vi "AppMenuSelection.vi"(8 "error in (no error)":errorcluster, 10 "Menu Selection in":string, 11 "xceRootNode in":refnum<class "xceRootNode.lvclass">) -> (0 "error out":errorcluster, 1 "New Message":string, 2 "Menu Selection out":string, 3 "xceRootNode out":refnum<class "xceRootNode.lvclass">)   [LabVIEW 2013, in "xceRootNode.lvclass"]
doc: "Processes the action related to the application level menu selection. For instance used when the user chooses \"File->Save\""
uses:
  xceRootNode.lvclass
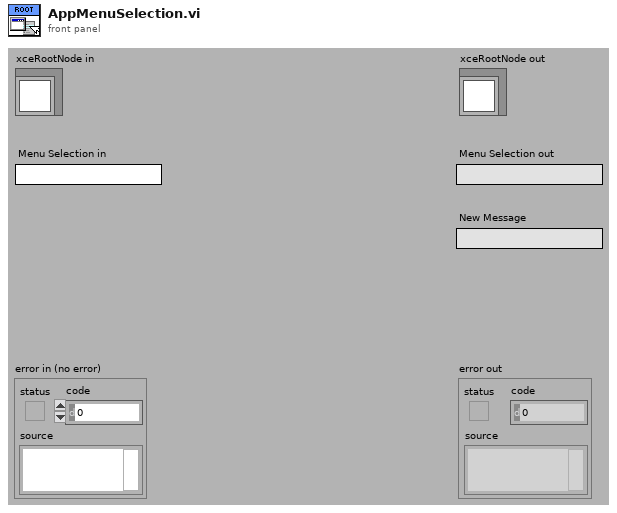
[diagram p1: front panel]
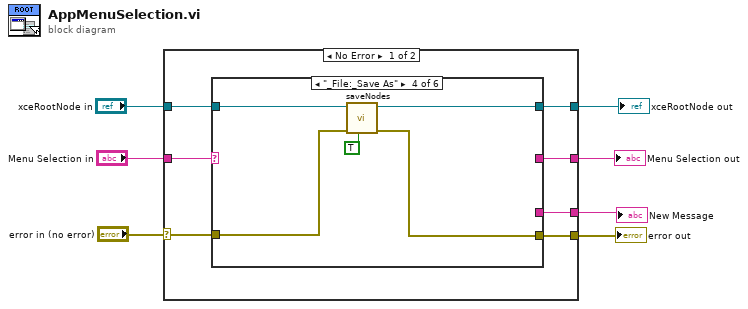
[diagram p0: block diagram]
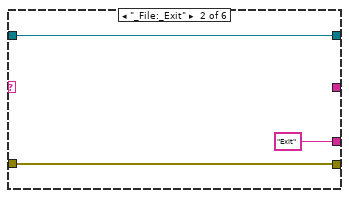
[diagram p3: hidden frame]
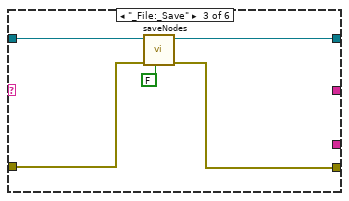
[diagram p4: hidden frame]
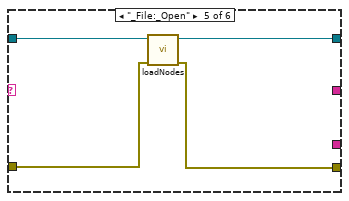
[diagram p5: hidden frame]
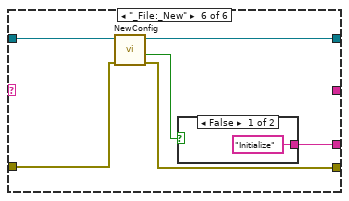
[diagram p6: hidden frame]
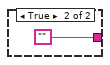
[diagram p7: hidden frame]
diagram:
  n1 = case shown="No Error" "error in (no error)" {
    selector: "error in (no error)" -> [w9 w44]
    tunnel: [w8 w44] -> w6
    tunnel: [w10 w43] -> w4
    tunnel: "xceRootNode in" -> [w11 w43]
    tunnel: "Menu Selection in" -> [w14 _]
    tunnel: [w13 _] -> w2
    tunnel: [w12 _] -> w1
    frame No Error {
      n2 = case shown="\"_File:_Save As\"" w14 {
        selector: w14 -> [w17 _ _ _ _ _]
        tunnel: [_ "Exit" _ _ _ w36] -> w13
        tunnel: [w17 _ _ _ _ _] -> w12
        tunnel: w11 -> [w15 w19 w25 w30 w34 w40]
        tunnel: [w15 w19 w24 w29 w33 w39] -> w10
        tunnel: w9 -> [w16 w18 w23 w28 w32 w38]
        tunnel: [w16 w18 w22 w27 w31 w35] -> w8
        frame Default {
        }
        frame "_File:_Exit" {
        }
        frame "_File:_Save" {
          n3 = call "saveNodes.vi"("Save As"=FALSE, "error in (no error)"=w23, "xceRootNode in"=w25) -> ("error out"=w22:errorcluster, "xceRootNode out"=w24:refnum<class "xceRootNode.lvclass">)  [unwired: 6 in, 1 out]
        }
        frame "_File:_Save As" {
          n4 = call "saveNodes.vi"("Save As"=TRUE, "error in (no error)"=w28, "xceRootNode in"=w30) -> ("error out"=w27:errorcluster, "xceRootNode out"=w29:refnum<class "xceRootNode.lvclass">)  [unwired: 6 in, 1 out]
        }
        frame "_File:_Open" {
          n5 = call "loadNodes.vi"("error in (no error)"=w32, "xceRootNode in"=w34) -> ("error out"=w31:errorcluster, "xceRootNode out"=w33:refnum<class "xceRootNode.lvclass">)  [unwired: 7 in, 1 out]
        }
        frame "_File:_New" {
          n6 = call "NewConfig.vi"("error in (no error)"=w38, "xceRootNode in"=w40) -> ("error out"=w35:errorcluster, "cancelled"=w37:bool, "xceRootNode out"=w39:refnum<class "xceRootNode.lvclass">)  [unwired: 7 in]
          n7 = case shown="False" w37 {
            tunnel: ["Initialize" ""] -> w36
            frame False {
            }
            frame True {
            }
          }
        }
      }
    }
    frame Error {
    }
  }
  "error out" <- w6
  "xceRootNode out" <- w4
  "Menu Selection out" <- w1
  "New Message" <- w2
